vi "Set GFG variable - Example.vi"() -> ()   [LabVIEW 2012]
doc: "SciScan 1.2 160622"
panel:
  in  "posX":dbl
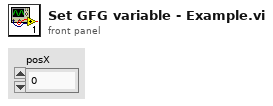
[diagram p1: front panel]
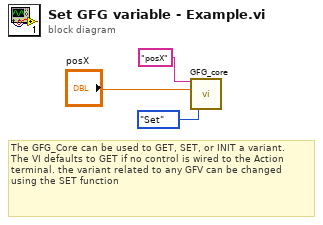
[diagram p0: block diagram]
diagram:
  # "The GFG_Core can be used to GET, SET, or INIT a variant. \nThe VI defaults to GET if no control is wired to the Action \nterminal. the variant related to any GFV can be changed\nusing the SET function"
  n1 = call "GFG_core.vi"("Variable Name in"="posX", "Variant in"="posX", "Action"=enum16{"Init", "Set", "Get"}."Set") -> ()  [unwired: 10 in, 7 out]
